vi "Read Values from System.vi"(8 "error in (no error)":errorcluster, 10 "Data In":dbl[](array[numeric]), 11 "Data References":T1[](array[typedef]) format="%.0x") -> (0 "error out":errorcluster, 2 "Data Out":dbl[](array[numeric]))   [LabVIEW 2021]
uses:
  <vilib>/NI VeriStand/Custom Device API/Data Reference.ctl
  <vilib>/NI VeriStand/Custom Device API/Global Data Refs.vi
  <vilib>/NI VeriStand/Custom Device API/Custom Device API.lvlib
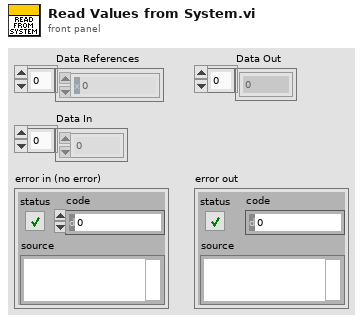
[diagram p1: front panel]
types:
  T1 = typedef "Custom Device API.lvlib/Data Reference.ctl" = i32
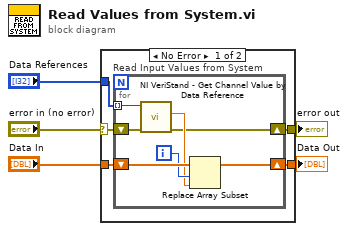
[diagram p0: block diagram]
diagram:
  n1 = case shown="No Error" "error in (no error)" {
    selector: "error in (no error)" -> [w10 w19]
    tunnel: "Data In" -> [w9 w18]
    tunnel: "Data References" -> [w8 _]
    tunnel: [w7 w19] -> w2
    tunnel: [w6 w18] -> w1
    frame No Error {
      n2 = for "Read Input Values from System" {
        shift-right: [w12] -> w7
        shift-left: w10 -> [w17]
        shift-right: [w15] -> w6
        shift-left: w9 -> [w16]
        tunnel: w8 -> [w11] mode=indexing
        i -> [w14]
        n3 = call <vilib>:"NI VeriStand - Get Channel Value by Data Reference.vi"("error in (no error)"=w17, "Data Reference in"=w11) -> ("error out"=w12:errorcluster, "Value"=w13:dbl)  [unwired: 8 out]
        n4 = Replace Array Subset(array=w16, new element=w13, index=w14) -> (w15:dbl[])
      }
    }
    frame Error {
    }
  }
  "error out" <- w2
  "Data Out" <- w1
